vi "Write Session Value.vi"(8 "error in (no error)":errorcluster, 9 "Value":string, 10 "Name":string, 11 "Processing in":refnum<class "Processing.lvclass">) -> (0 "error out":errorcluster, 2 "Value Replaced?":bool, 3 "Processing out":refnum<class "Processing.lvclass">)   [LabVIEW 2020, in "HTTP Server.lvlib" / "Processing.lvclass"]
uses:
  Processing.lvclass
  Processing.lvclass/Processing.ctl
  Session/Session.lvclass
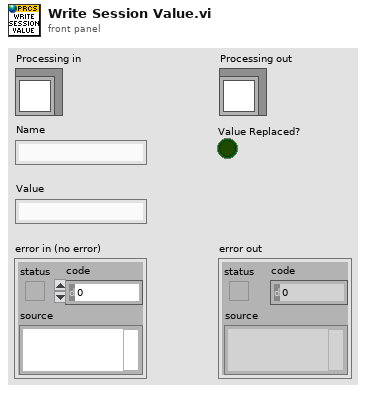
[diagram p1: front panel]
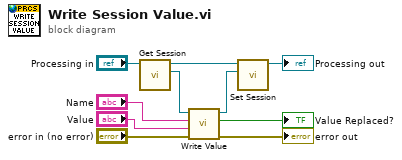
[diagram p0: block diagram]
diagram:
  n1 = call "Get Session.vi"("Processing in"="Processing in") -> ("Session"=w6:refnum<class "Session.lvclass">, "Processing out"=w5:refnum<class "Processing.lvclass">)  [unwired: 9 in]
  n2 = call "Write Value.vi"("error in (no error)"="error in (no error)", "Value"="Value", "Name"="Name", "Session in"=w6) -> ("error out"=→"error out":errorcluster, "Value Replaced?"=→"Value Replaced?":bool, "Session out"=w4:refnum<class "Session.lvclass">)  [unwired: 5 in]
  n3 = call "Set Session.vi"("Session"=w4, "Processing in"=w5) -> ("Processing out"=→"Processing out":refnum<class "Processing.lvclass">)  [unwired: 9 in]
